vi "Get ROI Area.vi"(8 "Error In":errorcluster, 11 "ROI Descriptor":T1 {"Contours"."Type" items=["No Selection", "Point", "Line", "Rectangle", "Oval", "Polygon", "Freehand Region", "Annulus", "Unused2", "Unused3", "Broken Line", "Freehand Line", "Rotated Rectangle"]}) -> (0 "Error Out":errorcluster, 3 "Number of Pixels":u32)   [LabVIEW 2021, in "Image.lvlib"]
uses:
  Image.lvlib
  <vilib>/vision/NI_Vision_Development_Module.lvlib
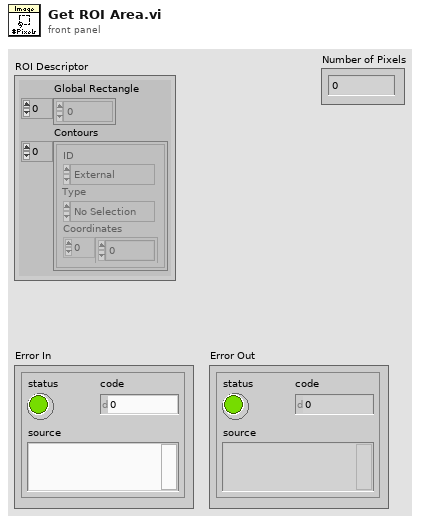
[diagram p1: front panel]
types:
  T1 = typedef "ROI Descriptor" = cluster{"Global Rectangle":i32[], "Contours":cluster{"ID":enum32{"External", "Internal"}, "Type":u32, "Coordinates":i32[]}[]}
  T2 = typedef "IMAQ Image.ctl" = refnum<image>
  T3 = cluster{"histogram":u32[], "Minimal Value":sgl, "Maximal Value":sgl, "Starting Value":sgl, "Interval Width":sgl, "Mean Value":sgl, "Standard  Variation":sgl, "Area (pixels)":i32}
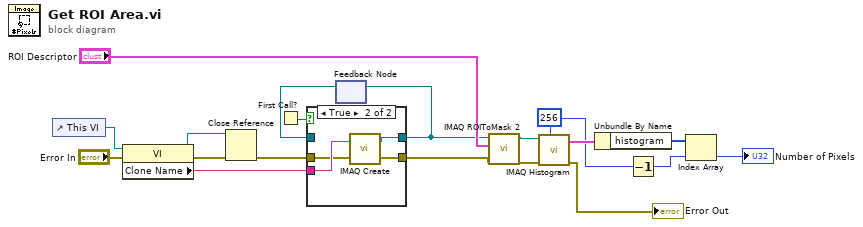
[diagram p0: block diagram]
diagram:
  w11 = 256 ("Number of Classes")
  n1 = control-ref of="This VI"() -> (w9:refnum<vi>)
  n2 = property class="VI"(reference=w9, error in="Error In") -> (reference out=w5:refnum<vi>, error out=w6:errorcluster, "Clone Name"=w7:string)
  n3 = Close Reference(reference=w5, error in (no error)=w6) -> (error out=w4:errorcluster)
  n4 = First Call?() -> (First Call?: T/F=w3:bool)
  n5 = feedback #1() -> (w2:T2)  [unwired: 1 in]
  n6 = case shown="True" w3 {
    tunnel: [w21 w25] -> w18
    tunnel: [w20 w24] -> w1
    tunnel: w7 -> [_ w23]
    tunnel: w4 -> [w21 w22]
    tunnel: w2 -> [w20 _]
    frame False {
    }
    frame True {
      n7 = call "IMAQ Create"("Image Name"=w23, "error in (no error)"=w22) -> ("New Image"=w24:T2, "error out"=w25:errorcluster)  [unwired: 3 in]
    }
  }
  n8 = feedback-in #1(w1) -> ()
  n9 = call "IMAQ ROIToMask 2"("error in (no error)"=w18, "ROI Descriptor"="ROI Descriptor", "Image"=w1) -> ("error out"=w16:errorcluster, "Image Out"=w15:T2)  [unwired: 6 in, 1 out]
  n10 = call "IMAQ Histogram"("Number of Classes"=w11, "error in (no error)"=w16, "Image"=w15) -> ("error out"=→"Error Out":errorcluster, "Histogram Report"=w17:T3)  [unwired: 7 in]
  n11 = Unbundle By Name(w17) -> ("histogram"=w13:u32[])
  n12 = Decrement(x=w11) -> (x-1=w10:i32)
  n13 = Index Array(array=w13, index=w10) -> (element=→"Number of Pixels":u32)
